vi "Synchio.Initialize.vi"(1 "AO Task":tag[](array[tag]), 2 "AI task":tag[](array[tag]), 8 "error in (no error)":errorcluster, 10 "AI/AO Config":T1={"AI Configuration"=[], "AO Configuration"=[], "sampling info"={"Fs"=0.0, "#s"=0.0}, "AO"={"AO amp (V)"=[0.1, 0.09, 0.08, 0.07, 0.06, 0.05, 0.04, 0.03], "AO DC (V)"=[0.0, 0.0, 0.0, 0.0, 0.0, 0.0, 0.0, 0.0], "AO f (Hz)"=[13.0, 13.0, 13.0, 13.0, 13.0, 13.0, 13.0, 13.0], "AO phi (deg)"=[0.0, 0.0, 0.0, 0.0, 0.0, 0.0, 0.0, 0.0], "function"=[enum."Sine Wave", enum."Sine Wave", enum."Sine Wave", enum."Sine Wave", enum."Sine Wave", enum."Sine Wave", enum."Sine Wave", enum."Sine Wave"]}} {"AO"."AO DC (V)" format="%#_6p"; "AO"."AO amp (V)" format="%#_6p"}, 11 "SynchIO in":refnum<class "SynchIO.lvclass">) -> (0 "error out":errorcluster, 3 "SynchIO out":refnum<class "SynchIO.lvclass">)   [LabVIEW 2016, in "SynchIO.lvclass"]
uses:
  SynchIO.lvclass
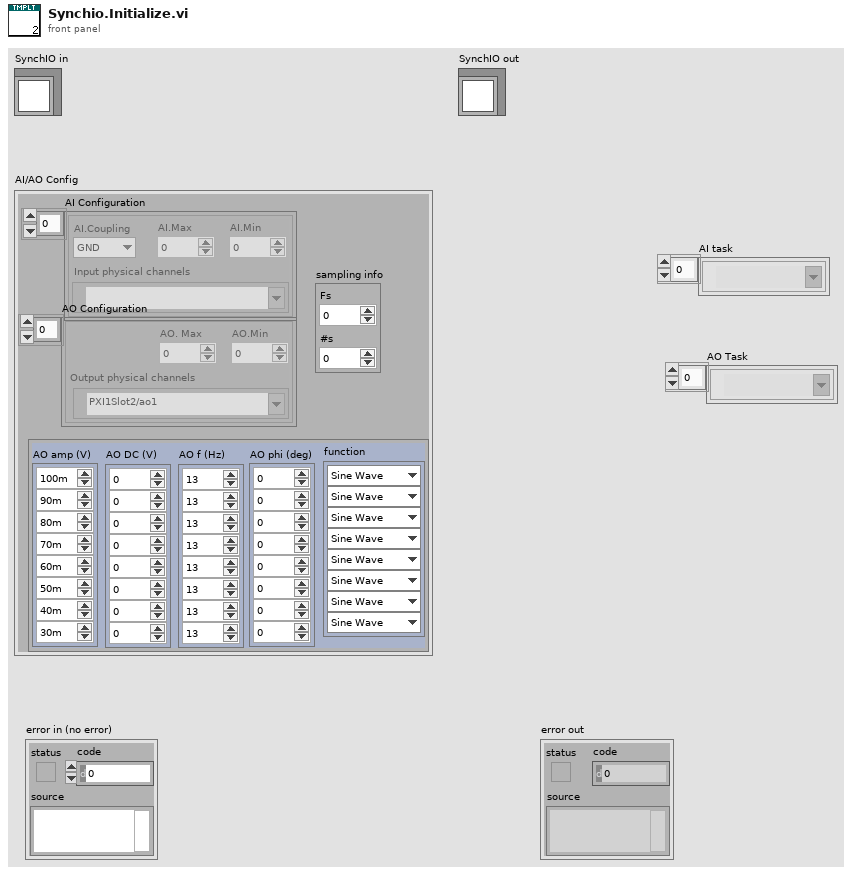
[diagram p1: front panel]
types:
  T1 = cluster{"AI Configuration":cluster{"AI.Coupling":enum16{"AC", "DC", "GND"}, "AI.Max":dbl, "AI.Min":dbl, "Input physical channels":tag}[], "AO Configuration":cluster{"Output physical channels":tag, "AO. Max":dbl, "AO.Min":dbl}[], "sampling info":cluster{"Fs":dbl, "#s":dbl}, "AO":cluster{"AO amp (V)":dbl[], "AO DC (V)":dbl[], "AO f (Hz)":dbl[], "AO phi (deg)":dbl[], "function":enum16{"Sine Wave", "Triangle Wave", "Square Wave", "Sawtooth Wave"}[]}}
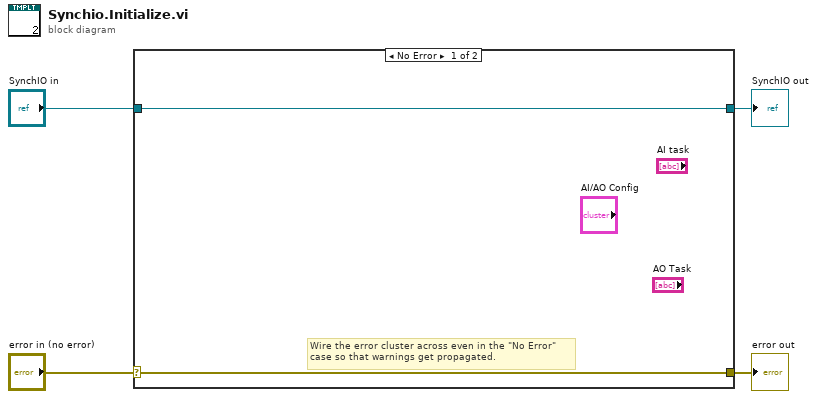
[diagram p0: block diagram]
diagram:
  n1 = case shown="No Error" "error in (no error)" {
    selector: "error in (no error)" -> [w5 w8]
    tunnel: [w5 w8] -> w3
    tunnel: [w6 w7] -> w1
    tunnel: "SynchIO in" -> [w6 w7]
    frame No Error {
      # "Wire the error cluster across even in the \"No Error\"\ncase so that warnings get propagated."
    }
    frame Error {
    }
  }
  "error out" <- w3
  "SynchIO out" <- w1
